vi "CRYMain Init.vi"(6 "This Application":refnum<vi>, 8 "Menu Refnum":refnum<k9>, 9 "Main View SubPanel":refnum<vi>, 10 "Pane":refnum<vi>, 11 "Main VI Ref":refnum<vi>) -> ()   [LabVIEW 2013]
uses:
  CRYMainGlobal.vi
  CRYSystem/Calibration/SubVI/CRYCal Global.vi
  CRYSystem/Task Sequence/CRYProject Run Control Global.vi
  CRYWindow/SubVI/CRYMain Sub Window Global.vi
  CRYProject/CRYProject Editor Global.vi
panel:
  in  "VI Refnum":refnum<vi>
  out "error out":errorcluster
  in  "error in (no error)":errorcluster
  # "Main Init."
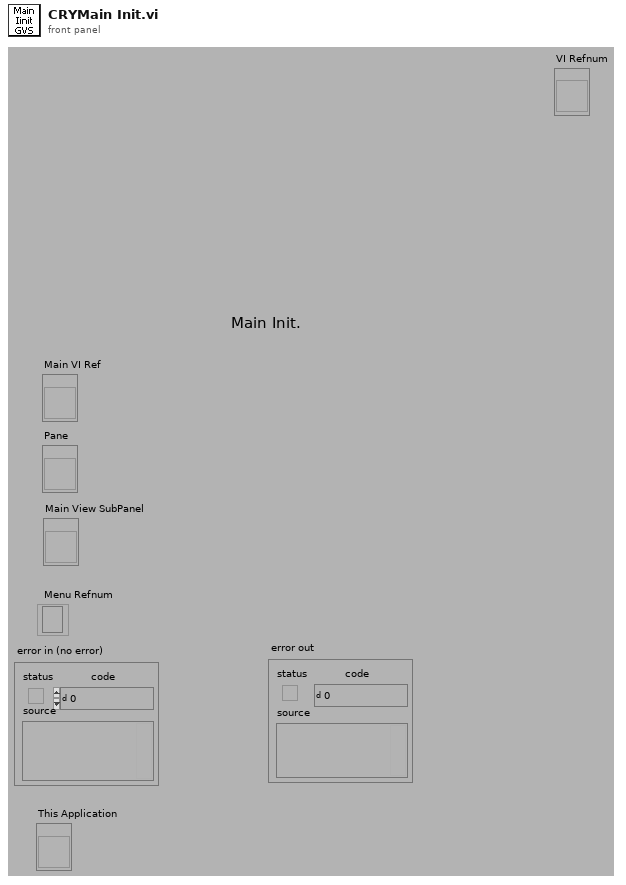
[diagram p1: front panel]
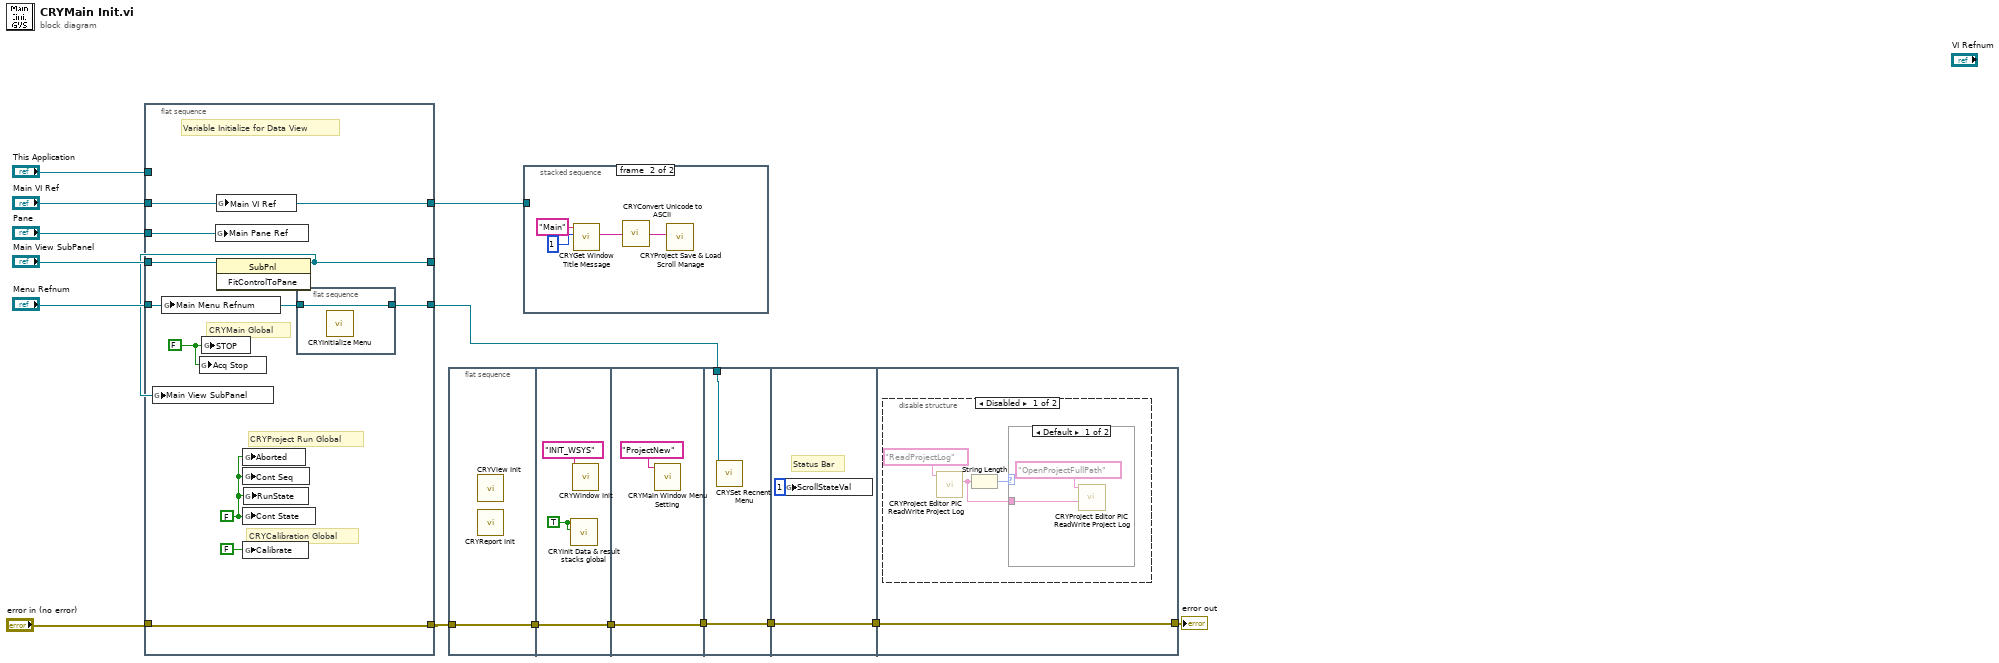
[diagram p0: block diagram]
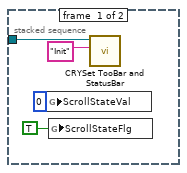
[diagram p2: hidden frame]
diagram:
  n1 = flat-sequence {
    tunnel: [w25] -> w10
    tunnel: "Main View SubPanel" -> [w24]
    tunnel: "error in (no error)" -> [w25]
    tunnel: "Main VI Ref" -> [w22]
    tunnel: "Menu Refnum" -> [w17]
    tunnel: "Pane" -> [w23]
    tunnel: [w22] -> w8
    tunnel: [w21] -> _
    tunnel: [w16] -> w5
    tunnel: "This Application" -> [_]
    frame #0 {
      w18 = FALSE ("STOP")
      w20 = FALSE ("STOP")
      # "CRYCalibration Global"
      # "CRYProject Run Global"
      # "CRYMain Global"
      # "Variable Initialize for Data View"
      n2 = global write "CRYMain Sub Window Global.vi" "Main Menu Refnum"(w17) -> ()
      n3 = global write "CRYMainGlobal.vi" "Acq Stop"(w20) -> ()
      n4 = global write "CRYMainGlobal.vi" "STOP"(w20) -> ()
      n5 = global write "CRYMain Sub Window Global.vi" "Main Pane Ref"(w23) -> ()
      n6 = global write "CRYMain Sub Window Global.vi" "Main VI Ref"(w22) -> ()
      n7 = invoke class="SubPnl" method="FitControlToPane"(reference=w24) -> (reference out=w21:refnum<vi>)  [unwired: 2 in, 2 out]
      n8 = global write "CRYMain Sub Window Global.vi" "Main View SubPanel"(w21) -> ()
      n9 = global write "CRYProject Run Control Global.vi" "Aborted"(w18) -> ()
      n10 = global write "CRYProject Run Control Global.vi" "Cont Seq"(w18) -> ()
      n11 = global write "CRYProject Run Control Global.vi" "Cont State"(w18) -> ()
      n12 = global write "CRYCal Global.vi" "Calibrate"(FALSE ("STOP")) -> ()
      n13 = global write "CRYProject Run Control Global.vi" "RunState"(w18) -> ()
      n14 = flat-sequence {
        tunnel: w17 -> [w26]
        tunnel: [w26] -> w16
        frame #0 {
          n15 = call "CRYInitialize Menu.vi"() -> ()  [unwired: 12 in]
        }
      }
    }
  }
  n16 = flat-sequence {
    tunnel: [w27] -> w2
    tunnel: w10 -> [w27]
    tunnel: [w30] -> w3
    tunnel: w2 -> [w30]
    tunnel: w3 -> [w32]
    tunnel: [w32] -> w7
    tunnel: w7 -> [w34]
    tunnel: [w34] -> w6
    tunnel: w5 -> [w33]
    tunnel: w6 -> [w36]
    tunnel: [w36] -> w4
    tunnel: [w37] -> w9
    tunnel: w4 -> [w37]
    frame #0 {
      n17 = call "CRYView Init.vi"() -> ()  [unwired: 12 in]
      n18 = call "CRYReport Init.vi"() -> ()  [unwired: 12 in]
    }
    frame #1 {
      w28 = TRUE ("Pause")
      n19 = call "CRYInit Data & result stacks global.vi"("Pause Proc"=w28, "Init?"=w28) -> ()  [unwired: 10 in]
      n20 = call "CRYWindow Init.vi"("sAction"="INIT_WSYS") -> ()  [unwired: 11 in]
    }
    frame #2 {
      n21 = call "CRYMain Window Menu Setting.vi"("sAction"="ProjectNew") -> ()  [unwired: 11 out]
    }
    frame #3 {
      n22 = call "CRYSet Recnent Menu.vi"("Main Menu Refnum in"=w33) -> ()  [unwired: 1 in, 10 out]
    }
    frame #4 {
      # "Status Bar"
      n23 = global write "CRYProject Editor Global.vi" "ScrollStateVal"(u8 1 ("ScrollStateVal")) -> ()
    }
    frame #5 {
      n24 = disable-structure shown="Disabled" {
        frame Disabled {
          n25 = call "CRYProject Editor PIC ReadWrite Project Log.vi"("sAction"="ReadProjectLog") -> ("sData_Out"=w38:string)  [unwired: 9 in, 1 out]
          n26 = String Length(string=w38) -> (length=w39:i32)
          n27 = case shown="Default" w39 {
            tunnel: w38 -> [w41 _]
            frame Default {
              n28 = call "CRYProject Editor PIC ReadWrite Project Log.vi"("sData"=w41, "sAction"="OpenProjectFullPath") -> ()  [unwired: 8 in, 2 out]
            }
            frame 0 {
            }
          }
        }
        frame Enabled {
        }
      }
    }
  }
  n29 = stacked-sequence {
    tunnel: w8 -> [w44 _]
    frame #0 {
      n30 = global write "CRYProject Editor Global.vi" "ScrollStateVal"(u8 0 ("ScrollStateVal")) -> ()
      n31 = global write "CRYProject Editor Global.vi" "ScrollStateFlg"(TRUE ("ScrollStateFlg")) -> ()
      n32 = call "CRYSet TooBar and StatusBar.vi"("Type"="Init", "MainVI Ref In"=w44) -> ()  [unwired: 2 in, 8 out]
    }
    frame #1 {
      n33 = call "CRYGet Window Title Message.vi"("No"=1, "Kind"="Main") -> ("Unicode String"=w48:string)  [unwired: 4 in, 5 out]
      n34 = call "CRYConvert Unicode to ASCII.vi"("Unicode"=w48) -> ("ASCII"=w47:string)  [unwired: 4 in]
      n35 = call "CRYProject Save & Load Scroll Manage.vi"("StateLabel"=w47) -> ()  [unwired: 1 in, 10 out]
    }
  }
  "error out" <- w9
